vi "Test_Pfeiffer.vi"() -> ()   [LabVIEW 2016]
uses:
  <vilib>/httpClient/POSTBuffer.vi
  <vilib>/httpClient/LabVIEWHTTPClient.lvlib
panel:
  in  "stop":bool
  out "Waveform Chart":dbl[](graph)
  in  "Address":string="10.0.1.201"
  out "headers":string
  out "body":string
  out "error out":errorcluster
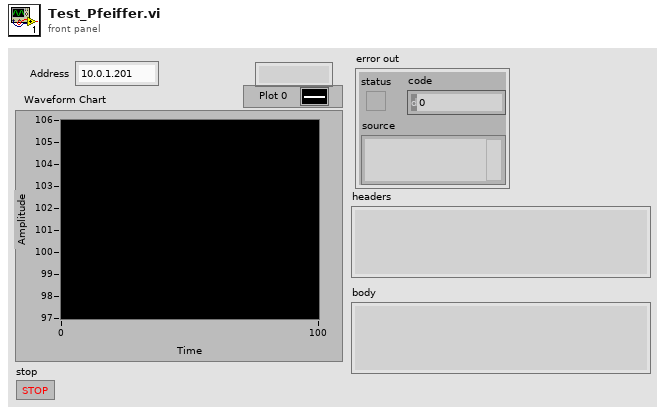
[diagram p1: front panel]
types:
  T1 = cluster{"Addr":i32[], "Kind":string[], "Pressure":dbl[]}
  T2 = typedef "LabVIEWHTTPClient.lvlib/ClientHandle.ctl" = refnum<k1>
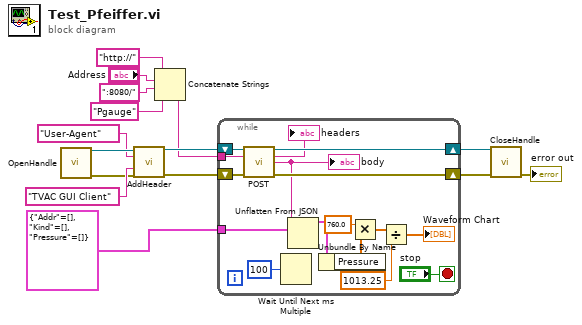
[diagram p0: block diagram]
diagram:
  n1 = call <vilib>:"OpenHandle.vi"() -> ("client handle out"=w15:T2, "error out"=w12:errorcluster)  [unwired: 14 in]
  n2 = call <vilib>:"AddHeader.vi"("client handle"=w15, "header"="User-Agent", "value"="TVAC GUI Client", "error in (no error)"=w12) -> ("client handle out"=w10:T2, "error out"=w11:errorcluster)  [unwired: 10 in]
  n3 = Concatenate Strings("http://" ("url"), "Address", ":8080/" ("url"), "Pgauge" ("url")) -> (w5:string)
  n4 = while {
    tunnel: w5 -> [w26]
    tunnel: T1 {"Addr"=[], "Kind"=[], "Pressure"=[]} -> [w24]
    shift-right: [w28] -> w7
    shift-left: w11 -> [w31]
    shift-right: [w29] -> w8
    shift-left: w10 -> [w30]
    stop <- "stop" stop-if-true
    n5 = call-poly <vilib>:"POST.vi"("client handle"=w30, "url"=w26, "error in (no error)"=w31) -> ("client handle out"=w29:T2, "headers"=→"headers":string, "body"=w25:string, "error out"=w28:errorcluster)  [unwired: 9 in]
    "body" <- w25
    n6 = Wait Until Next ms Multiple(millisecond multiple=u32 100) -> ()  [unwired: 1 out]
    n7 = Unflatten From JSON(JSON string=w25, type and defaults=w24) -> (value=w23:T1)  [unwired: 5 in, 1 out]
    n8 = Unbundle By Name(w23) -> ("Pressure"=w22:dbl[])
    n9 = Multiply(x=760.0, y=w22) -> (x*y=w21:dbl[])
    n10 = Divide(x=w21, y=1013.25) -> (x/y=→"Waveform Chart":dbl[])
  }
  n11 = call <vilib>:"CloseHandle.vi"("client handle"=w8, "error in (no error)"=w7) -> ("error out"=→"error out":errorcluster)  [unwired: 13 in]
